vi "MTM2_getNextSample_netForcesTotal.vi"(8 "error in (no error)":errorcluster, 11 "netForcesTotal_Ctl":T1) -> (0 "error out":errorcluster, 2 "function return":i32, 3 "netForcesTotal_Ctl out":T1)   [LabVIEW 2018, in "SALLV_MTM2.lvlib"]
doc: "int MTM2_shm_getNextSample_netForcesTotalLV(MTM2_netForcesTotalLV *netForcesTotal_Ctl );"
uses:
  DataTypes/netForcesTotal.ctl
  SALLV_MTM2.lvlib
  SALLV_MTM2.so
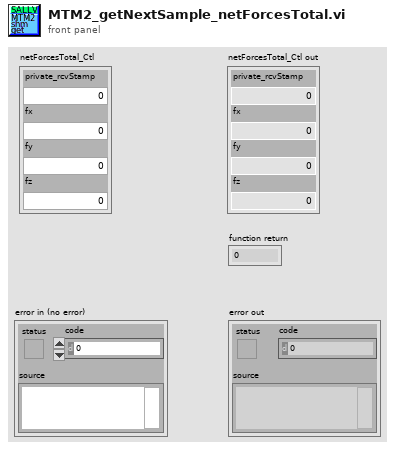
[diagram p1: front panel]
types:
  T1 = typedef "SALLV_MTM2.lvlib/netForcesTotal.ctl" = cluster{"private_rcvStamp":dbl, "fx":dbl, "fy":dbl, "fz":dbl}
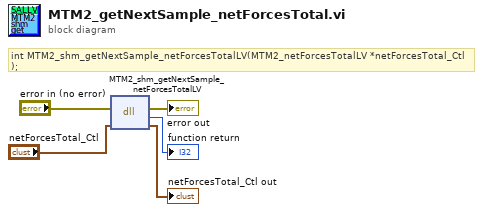
[diagram p0: block diagram]
diagram:
  # "int MTM2_shm_getNextSample_netForcesTotalLV(MTM2_netForcesTotalLV *netForcesTotal_Ctl );"
  n1 = dll-call lib="home/ttsai/Documents/salLabviewApi/SALLV_MTM2/SALLV_MTM2.*" fn="MTM2_shm_getNextSample_netForcesTotalLV"(error in="error in (no error)", "netForcesTotal_Ctl"="netForcesTotal_Ctl") -> (error out=→"error out":errorcluster, →"function return":i32, "netForcesTotal_Ctl"=→"netForcesTotal_Ctl out":T1)  [unwired: 2 in, 1 out]
